vi "ep_Digital Data to U16 (Waveform).vi"(8 "error in":errorcluster, 11 "digital signal":waveform(u16)[](array[waveform])) -> (0 "error out":errorcluster, 3 "U16 digital data":u16[][](array[numeric])=[[0, 2], [0, 17]])   [LabVIEW 2011, in "NI_EP_COMTRADE.lvlib"]
uses:
  <vilib>/addons/Electrical Power/File IO/NI_EP_COMTRADE.lvlib
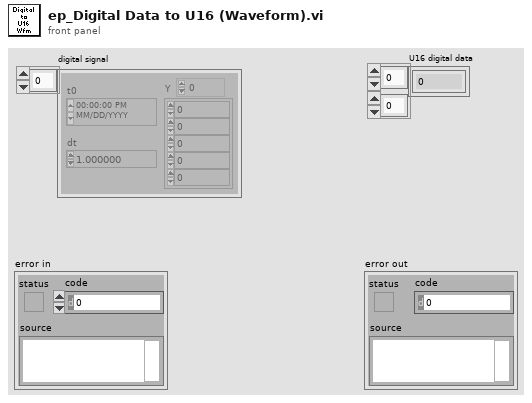
[diagram p1: front panel]
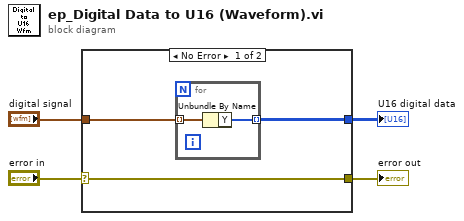
[diagram p0: block diagram]
diagram:
  n1 = case shown="No Error" "error in" {
    selector: "error in" -> [w5 w10]
    tunnel: "digital signal" -> [w7 _]
    tunnel: [w5 w10] -> w2
    tunnel: [w6 _] -> w1
    frame No Error {
      n2 = for {
        tunnel: w7 -> [w9] mode=indexing
        tunnel: [w8] -> w6 mode=indexing
        n3 = Unbundle By Name(w9) -> ("Y"=w8:u16[])
      }
    }
    frame Error {
    }
  }
  "error out" <- w2
  "U16 digital data" <- w1
